vi "GraphClear.vi"(11 "Graph Reference Cluster":T1) -> ()   [LabVIEW 2014]
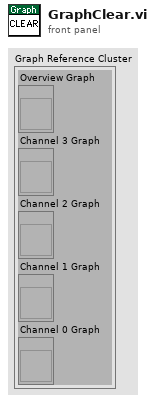
[diagram p1: front panel]
types:
  T1 = cluster{"Overview Graph":refnum<vi>, "Channel 3 Graph":refnum<vi>, "Channel 2 Graph":refnum<vi>, "Channel 1 Graph":refnum<vi>, "Channel 0 Graph":refnum<vi>}
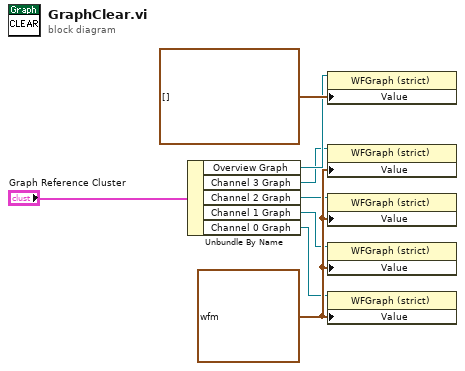
[diagram p0: block diagram]
diagram:
  w7 = waveform(dbl) {"t0"=timestamp(0 s since 1904-01-01), "dt"=1.0, "Y"=[]} ("Channel 0 Graph")
  n1 = Unbundle By Name("Graph Reference Cluster") -> ("Overview Graph"=w5:refnum<vi>, "Channel 3 Graph"=w4:refnum<vi>, "Channel 2 Graph"=w3:refnum<vi>, "Channel 1 Graph"=w2:refnum<vi>, "Channel 0 Graph"=w1:refnum<vi>)
  n2 = property on="Property Node" class="WFGraph (strict)"(reference=w5, "Value"=waveform(dbl)[] [] ("Overview Graph")) -> ()  [unwired: 1 in, 2 out]
  n3 = property on="Property Node" class="WFGraph (strict)"(reference=w4, "Value"=w7) -> ()  [unwired: 1 in, 2 out]
  n4 = property on="Property Node" class="WFGraph (strict)"(reference=w3, "Value"=w7) -> ()  [unwired: 1 in, 2 out]
  n5 = property on="Property Node" class="WFGraph (strict)"(reference=w2, "Value"=w7) -> ()  [unwired: 1 in, 2 out]
  n6 = property on="Property Node" class="WFGraph (strict)"(reference=w1, "Value"=w7) -> ()  [unwired: 1 in, 2 out]
